vi "Main.vi"(11 "Module Admin":refnum<class "Delacor_lib_QMH_Module Admin.lvclass">) -> ()   [LabVIEW 2018, in "Configuration.lvlib"]
doc: "This template is based off of the Queued Message Handler design pattern and the Queued Message Handler project template that ships with LabVIEW.\n\nThe main difference is that the queue is private to this module and communication between modules is performed via Broadcast and Request events.\n\nRequest events are wrapped in public API methods and are handled in the Event Handling Loop (EHL) of this VI. Any module can register for Broadcast events sent by this module. The EHL generates messages based on user interface actions.\n\nThe Message Handling Loop (MHL) processes messages generated by the EHL, or by other messages. The messages are string values, so new messages can be added easily to the Message Cases case structure in the MHL. Each message cluster can also provide an optional value for Message Data, which is a variant that can be converted to whatever message-specific data is required.\n_____\nBased on DQMH Project Template 6.0.0.91."
uses:
  Configuration.lvlib
  <vilib>/Delacor/Delacor QMH/Libraries/Module Admin_class/Delacor_lib_QMH_Module Admin.lvclass
  Module Data--cluster.ctl
  <vilib>/Delacor/Delacor QMH/Libraries/Message Queue_class/Delacor_lib_QMH_Message Queue.lvclass/Delacor_lib_QMH_Message Queue.ctl
  Stop Argument--cluster.ctl
  <vilib>/Delacor/Delacor QMH/Libraries/Module Admin_class/Delacor_lib_QMH_Module Admin.lvclass/Delacor_lib_QMH_Module Admin.ctl
  <vilib>/Utility/miscctls.llb/LVPointTypeDef.ctl
  <vilib>/Delacor/Delacor QMH/Libraries/Message Queue_class/Delacor_lib_QMH_Enqueue Message (Single).vi
  <vilib>/Delacor/Delacor QMH/Libraries/Module Admin_class/Delacor_lib_QMH_Get External Launch.vi
  <vilib>/Utility/error.llb/Error Cluster From Error Code.vi
  <vilib>/ErrorRing/Error Ring.xnode
  <vilib>/Delacor/Delacor QMH/Libraries/Message Queue_class/Delacor_lib_QMH_Message Queue.lvclass
panel:
  in  "OK":bool
  in  "Cancel":bool
  in  "# DUTs":string
  in  "ma SAP":string
  in  "Password":string
  in  "User":string
  out "error out":errorcluster
  out "Status":string
  in  "Simulate MHL Error":bool
  in  "Simulate EHL Error":bool
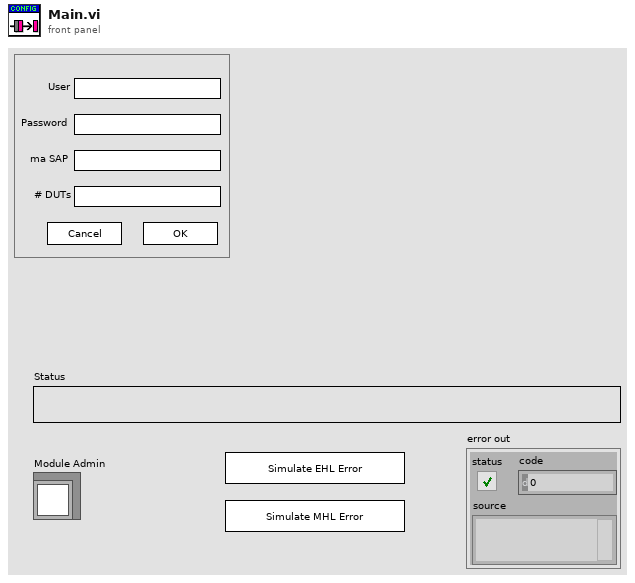
[diagram p1: front panel]
types:
  T1 = enum8{"Enabled", "Disabled", "Disabled and Grayed Out"}
  T2 = typedef "Configuration.lvlib/Request Events--cluster.ctl" = cluster{"Stop Module":refnum<user-event>, "Show Panel":refnum<user-event>, "Hide Panel":refnum<user-event>, "Get Module Execution Status":refnum<user-event>, "Show Diagram":refnum<user-event>}
  T3 = typedef "Configuration.lvlib/Module Data--cluster.ctl" = cluster{"Status":string}
  T4 = enum32{"invalid lock state", "Not Locked", "Locked (No Password)", "Password-protected"}
  T5 = typedef "Configuration.lvlib/Stop Argument--cluster.ctl" = cluster{"Origin":string, "Exit via Stop Module Req?":bool, "Wait for Module to stop?":bool}
  T6 = typedef "LVPointTypeDef.ctl" = cluster{"Horizontal":i16, "Vertical":i16}
  T7 = enum32{"Invalid", "Standard", "Closed", "Hidden", "Minimized", "Maximized"}
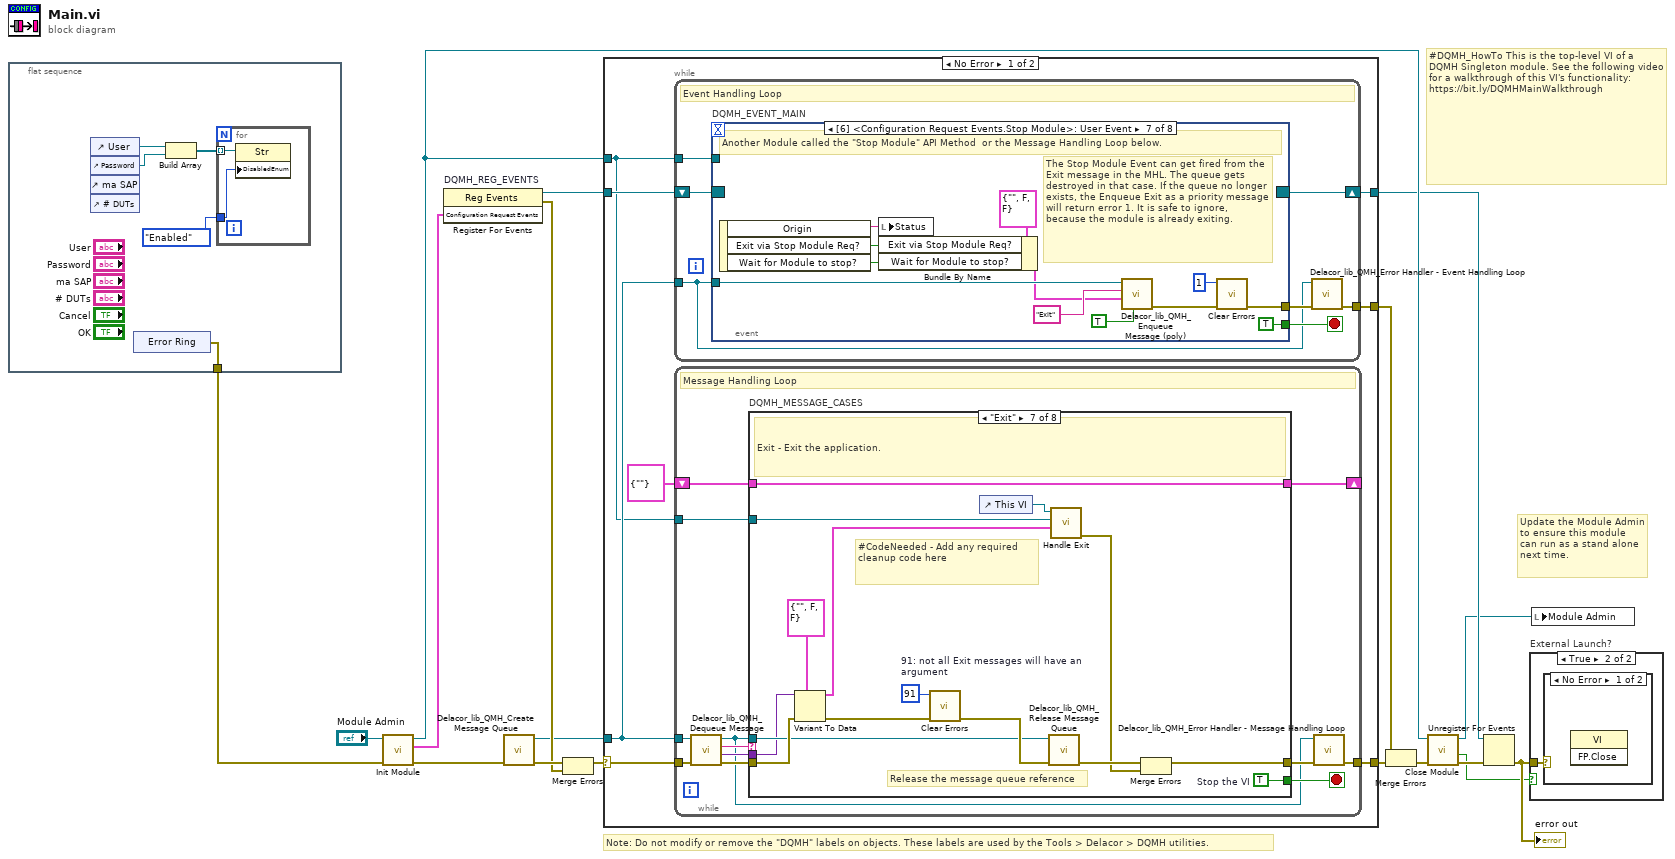
[diagram p0: block diagram]
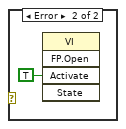
[diagram p3: hidden frame]
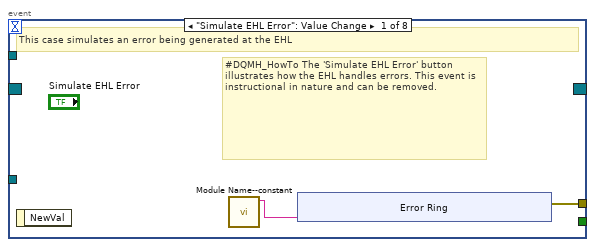
[diagram p4: hidden frame]
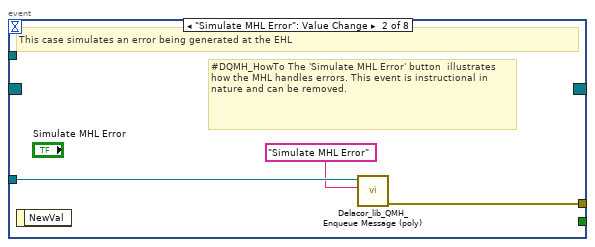
[diagram p5: hidden frame]
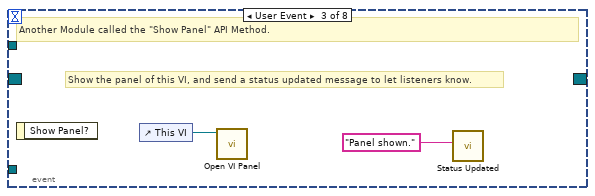
[diagram p6: hidden frame]
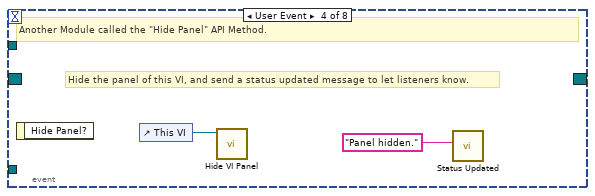
[diagram p7: hidden frame]
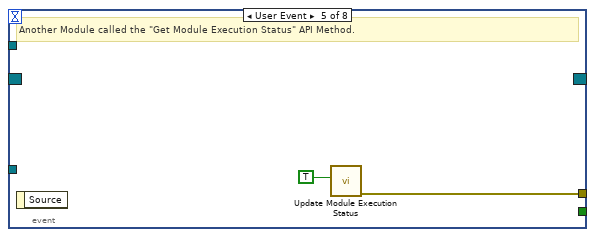
[diagram p8: hidden frame]
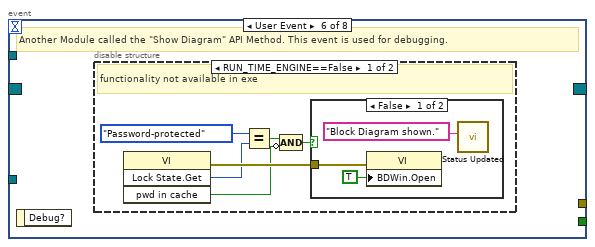
[diagram p9: hidden frame]
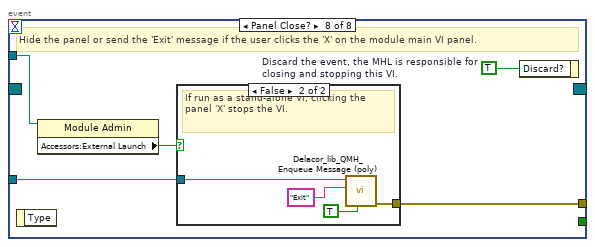
[diagram p12: hidden frame]
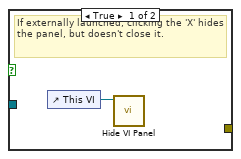
[diagram p13: hidden frame]
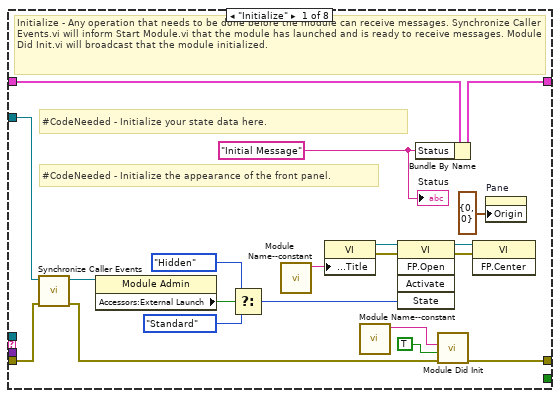
[diagram p14: hidden frame]
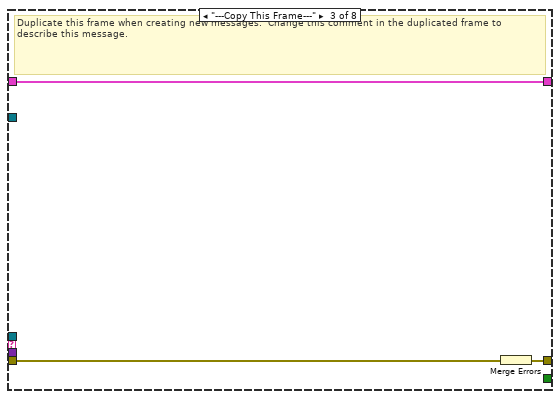
[diagram p16: hidden frame]
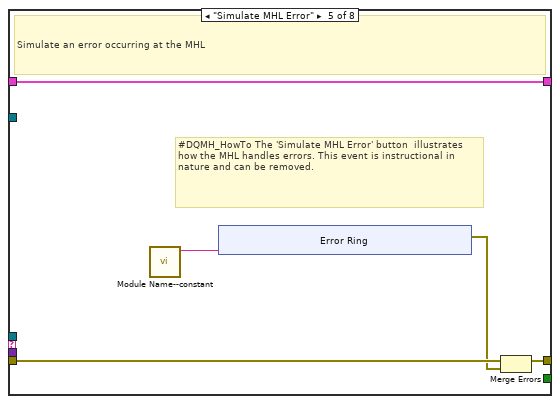
[diagram p18: hidden frame]
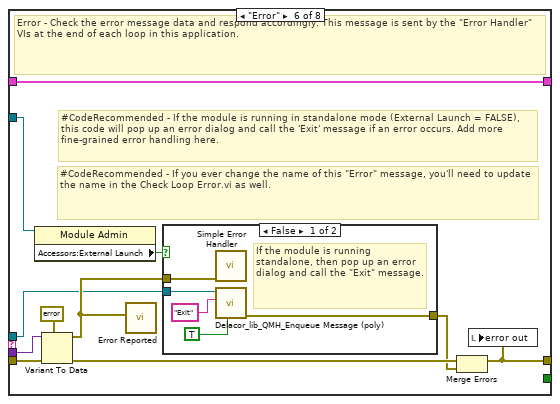
[diagram p19: hidden frame]
diagram:
  # "#DQMH_HowTo This is the top-level VI of a DQMH Singleton module. See the following video for a walkthrough of this VI's functionality: https://bit.ly/DQMHMainWalkthrough"
  # "Note: Do not modify or remove the \"DQMH\" labels on objects. These labels are used by the Tools > Delacor > DQMH utilities."
  # "Update the Module Admin to ensure this module can run as a stand alone next time."
  n1 = flat-sequence {
    tunnel: [w19] -> w1
    frame #0 {
      n2 = control-ref of="User"() -> (w22:refnum<vi>)
      n3 = control-ref of="Password"() -> (w21:refnum<vi>)
      n4 = control-ref of="ma SAP"() -> ()  [unwired: 1 out]
      n5 = control-ref of="# DUTs"() -> ()  [unwired: 1 out]
      n6 = xnode "Error Ring"() -> ("error out"=w19:errorcluster)
      n7 = Build Array(w22, w21) -> (w20:refnum<vi>[])
      n8 = for {
        tunnel: w20 -> [w26] mode=indexing
        tunnel: T1."Enabled" ("Disabled") -> [w25]
        n9 = property class="Str"(reference=w26, "DisabledEnum"=w25) -> ()  [unwired: 1 in, 2 out]
      }
    }
  }
  n10 = call "Init Module.vi"("error in (no error)"=w1, "Singleton Module Admin in"="Module Admin") -> ("error out"=w17:errorcluster, "Configuration Request Events"=w6:T2, "Singleton Module Admin out"=w9:refnum<class "Delacor_lib_QMH_Module Admin.lvclass">)  [unwired: 7 in]
  n11 = register-events "DQMH_REG_EVENTS"(w6) -> (reference out=w7:refnum<event-registration>, error out=w10:errorcluster)  [unwired: 2 in]
  n12 = call <vilib>:"Delacor_lib_QMH_Create Message Queue.vi"("error in"=w17) -> ("error out"=w12:errorcluster, "Message Queue"=w5:refnum<class "Delacor_lib_QMH_Message Queue.lvclass">)  [unwired: 9 in]
  n13 = Merge Errors(w12, w10) -> (w11:errorcluster)
  n14 = case shown="No Error" w11 {
    selector: w11 -> [w32 w189]
    tunnel: [w34 w188] -> w18
    tunnel: [w31 w194] -> w8
    tunnel: w7 -> [w29 w194]
    tunnel: w5 -> [w28 w187]
    tunnel: [w33 _] -> w15
    tunnel: w9 -> [w27 w190]
    frame No Error {
      n15 = while {
        tunnel: w28 -> [w35]
        shift-right: [w38] -> w31
        shift-left: w29 -> [w39]
        tunnel: [w40] -> w33
        tunnel: w27 -> [w36]
        stop <- w37 stop-if-true
        # "Event Handling Loop"
        n16 = event "DQMH_EVENT_MAIN" shown="[6] <Configuration Request Events.Stop Module>: User Event" {
          selector: w39 -> [_ _ _ _ _ _ _ _]
          dyn-events: [_ _ _ _ _ _ _ _] -> w38
          timeout: _ -> [_ _ _ _ _ _ _ _]
          tunnel: [_ _ _ _ _ _ TRUE ("Discard?") _] -> w37
          tunnel: w35 -> [_ w52 _ _ _ _ w76 w83]
          tunnel: [w43 w53 _ _ w59 _ w79 w85] -> w41
          tunnel: w36 -> [_ _ _ _ _ _ _ w82]
          event "Simulate EHL Error": Value Change {
            # "#DQMH_HowTo The 'Simulate EHL Error' button  illustrates how the EHL handles errors. This event is instructional in nature and can be removed."
            # "This case simulates an error being generated at the EHL"
            n17 = event-data() -> ()  [unwired: 1 in, 1 out]
            n18 = call "Module Name--constant.vi"() -> ("Module Name"=w42:string)  [unwired: 11 in]
            n19 = xnode "Error Ring"("parameter 0"=w42) -> ("error out"=w43:errorcluster)
          }
          event "Simulate MHL Error": Value Change {
            # "#DQMH_HowTo The 'Simulate MHL Error' button  illustrates how the MHL handles errors. This event is instructional in nature and can be removed."
            # "This case simulates an error being generated at the EHL"
            n20 = event-data() -> ()  [unwired: 1 in, 1 out]
            n21 = call-poly <vilib>:"Delacor_lib_QMH_Enqueue Message (poly).vi"("Message"="Simulate MHL Error", "Message Queue in"=w52) -> ("error out"=w53:errorcluster)  [unwired: 8 in, 1 out]
          }
          event User Event {
            # "Show the panel of this VI, and send a status updated message to let listeners know."
            # "Another Module called the \"Show Panel\" API Method."
            n22 = event-data() -> ()  [unwired: 1 in, 1 out]
            n23 = control-ref of="This VI"() -> (w55:refnum<vi>)
            n24 = call "Open VI Panel.vi"("VI"=w55) -> ()  [unwired: 10 in, 1 out]
            n25 = call "Status Updated.vi"("Status"="Panel shown." ("format string")) -> ()  [unwired: 10 in, 1 out]
          }
          event User Event {
            # "Hide the panel of this VI, and send a status updated message to let listeners know."
            # "Another Module called the \"Hide Panel\" API Method."
            n26 = event-data() -> ()  [unwired: 1 in, 1 out]
            n27 = control-ref of="This VI"() -> (w57:refnum<vi>)
            n28 = call "Hide VI Panel.vi"("VI"=w57) -> ()  [unwired: 10 in, 1 out]
            n29 = call "Status Updated.vi"("Status"="Panel hidden." ("format string")) -> ()  [unwired: 10 in, 1 out]
          }
          event User Event {
            # "Another Module called the \"Get Module Execution Status\" API Method."
            n30 = event-data() -> ()  [unwired: 1 in, 1 out]
            n31 = call "Update Module Execution Status.vi"("Running?"=TRUE) -> ("error out"=w59:errorcluster)  [unwired: 10 in]
          }
          event User Event {
            # "Another Module called the \"Show Diagram\" API Method. This event is used for debugging."
            n32 = event-data() -> ()  [unwired: 1 in, 1 out]
            n33 = disable-structure shown="RUN_TIME_ENGINE==False" {
              frame condition #0 (active) {
                # "functionality not available in exe"
                n34 = invoke class="VI" method="Lock State.Get"() -> (error out=w65:errorcluster, "Get Lock State"=w64:T4, "pwd in cache"=w61:bool)  [unwired: 4 in, 1 out]
                n35 = Equal?(x=T4."Password-protected", y=w64) -> (x = y?=w62:bool)
                n36 = Compound Arithmetic op=AND(w62, invert w61) -> (w60:bool)
                n37 = case shown="False" w60 {
                  tunnel: w65 -> [w68 _]
                  frame False {
                    n38 = property class="VI"(error in=w68, "BDWin.Open"=TRUE ("Block Diagram Window:Open")) -> ()  [unwired: 1 in, 2 out]
                    n39 = call "Status Updated.vi"("Status"="Block Diagram shown." ("format string")) -> ()  [unwired: 10 in, 1 out]
                  }
                  frame True {
                    # "Password-protected VI, and the password is not in the cache. Do not show the diagram."
                  }
                }
              }
              frame condition #1 {
              }
            }
          }
          event User Event {
            # "The Stop Module Event can get fired from the Exit message in the MHL. The queue gets destroyed in that case. If the queue no longer exists, the Enqueue Exit as a priority message will return error 1. It is safe to ignore, because the module is already exiting."
            # "Another Module called the \"Stop Module\" API Method  or the Message Handling Loop below."
            n40 = event-data() -> ("Origin"=w75:string, "Exit via Stop Module Req?"=w71:bool, "Wait for Module to stop?"=w70:bool)  [unwired: 1 in]
            n41 = local write "Status"(w75) -> ()
            n42 = Bundle By Name(cluster=T5 {"Origin"="", "Exit via Stop Module Req?"=FALSE, "Wait for Module to stop?"=FALSE} ("Stop Argument"), "Exit via Stop Module Req?"=w71, "Wait for Module to stop?"=w70) -> (w69:T5)
            n43 = call-poly <vilib>:"Delacor_lib_QMH_Enqueue Message (poly).vi"("Priority Message? (F)"=TRUE, "Message Data"=w69, "Message"="Exit", "Message Queue in"=w76) -> ("error out"=w80:errorcluster)  [unwired: 6 in, 1 out]
            n44 = call <vilib>:"Clear Errors.vi"("error in (no error)"=w80, "specific error code to clear (0: all)"=1) -> ("error out"=w79:errorcluster)  [unwired: 4 in, 1 out]
          }
          event Panel Close? {
            w84 = TRUE  # Discard the event, the MHL is responsible for closing and stopping this VI.
            # "Hide the panel or send the 'Exit' message if the user clicks the 'X' on the module main VI panel."
            n45 = event-data() -> ()  [unwired: 1 in, 1 out]
            n46 = property class="Module Admin"(reference=w82) -> ("Accessors:External Launch"=w81:bool)  [unwired: 1 in, 2 out]
            n47 = case shown="False" w81 {
              tunnel: w83 -> [_ w89]
              tunnel: [_ w90] -> w85
              frame True {
                # "If externally launched, clicking the 'X' hides the panel, but doesn't close it."
                n48 = control-ref of="This VI"() -> (w86:refnum<vi>)
                n49 = call "Hide VI Panel.vi"("VI"=w86) -> ()  [unwired: 10 in, 1 out]
              }
              frame False {
                # "If run as a stand-alone VI, clicking the panel 'X' stops the VI."
                n50 = call-poly <vilib>:"Delacor_lib_QMH_Enqueue Message (poly).vi"("Priority Message? (F)"=TRUE, "Message"="Exit", "Message Queue in"=w89) -> ("error out"=w90:errorcluster)  [unwired: 7 in, 1 out]
              }
            }
            n51 = event-data("Discard?"=w84) -> ()  [unwired: 1 in, 1 out]
          }
        }
        n52 = call-dynamic "Delacor_lib_QMH_Error Handler - Event Handling Loop.vi"("error in"=w41, "Message Queue in"=w35) -> ("dup error in"=w40:errorcluster)  [unwired: 8 in, 1 out]
      }
      n53 = while {
        tunnel: w28 -> [w93]
        shift-right: [w97] -> _
        shift-left: T3 {"Status"=""} ("Data Cluster") -> [w98]
        tunnel: w32 -> [w101]
        tunnel: [w99] -> w34
        tunnel: w27 -> [w91]
        stop <- w96 stop-if-true
        # "Message Handling Loop"
        n54 = call-dynamic "Delacor_lib_QMH_Dequeue Message.vi"("error in"=w101, "Message Queue in"=w93) -> ("error out"=w100:errorcluster, "Message Data"=w94:variant, "Message"=w95:string, "Message Queue out"=w92:refnum<class "Delacor_lib_QMH_Message Queue.lvclass">)  [unwired: 6 in]
        n55 = case "DQMH_MESSAGE_CASES" shown="\"Exit\"" w95 {
          selector: w95 -> [_ _ _ _ _ _ _ w174]
          tunnel: w92 -> [_ _ _ _ _ w144 w166 _]
          tunnel: w100 -> [w120 w124 w127 w129 w134 w151 w172 w176]
          tunnel: [w118 w124 w126 w129 w133 w147 w169 w177] -> w102
          tunnel: w98 -> [w109 w123 w125 w128 w131 w146 w165 w175]
          tunnel: [w108 w123 w125 w128 w131 w146 w165 w175] -> w97
          tunnel: [_ _ _ _ _ _ w164 _] -> w96
          tunnel: w94 -> [_ _ _ _ _ w145 w163 _]
          tunnel: w91 -> [w110 _ _ _ _ w143 w158 _]
          frame "Initialize" {
            w104 = "Initial Message" ("Initial Message")
            # "#CodeNeeded - Initialize the appearance of the front panel."
            # "#CodeNeeded - Initialize your state data here."
            # "Initialize - Any operation that needs to be done before the module can receive messages. Synchronize Caller Events.vi will inform Start Module.vi that the module has launched and is ready to receive messages. Module Did Init.vi will broadcast that the module initialized."
            n56 = call "Synchronize Caller Events.vi"("error in (no error)"=w120, "Singleton Module Admin in"=w110) -> ("error out"=w119:errorcluster, "Singleton Module Admin out"=w105:refnum<class "Delacor_lib_QMH_Module Admin.lvclass">)  [unwired: 8 in]
            n57 = property class="Module Admin"(reference=w105) -> ("Accessors:External Launch"=w114:bool)  [unwired: 1 in, 2 out]
            n58 = Select(t=T7."Hidden" ("State"), s=w114, f=T7."Standard" ("State")) -> (s? t:f=w111:T7)
            n59 = call "Module Name--constant.vi"() -> ("Module Name"=w117:string)  [unwired: 11 in]
            n60 = property class="VI"("Front Panel.Title"=w117) -> (reference out=w116:refnum<vi>, error out=w122:errorcluster)  [unwired: 2 in]
            n61 = call "Module Name--constant.vi"() -> ("Module Name"=w106:string)  [unwired: 11 in]
            n62 = invoke class="VI" method="FP.Open"(reference=w116, error in=w122, "State"=w111) -> (reference out=w115:refnum<vi>, error out=w121:errorcluster)  [unwired: 2 in, 3 out]
            n63 = Bundle By Name(cluster=w109, "Status"=w104) -> (w108:T3)
            n64 = call "Module Did Init.vi"("error in (no error)"=w119, "Initialized?"=TRUE, "Origin"=w106) -> ("error out"=w118:errorcluster)  [unwired: 8 in]
            n65 = invoke class="VI" method="FP.Center"(reference=w115, error in=w121) -> ()  [unwired: 1 in, 3 out]
            n66 = property on="Pane" class="Pane"("Origin"=T6 {"Horizontal"=0, "Vertical"=0}) -> ()  [unwired: 2 in, 2 out]
            "Status" <- w104
          }
          frame "---Module Specific---" {
            # "Separator -- The following cases handle messages specific to this Module."
          }
          frame "---Copy This Frame---" {
            # "Duplicate this frame when creating new messages.  Change this comment in the duplicated frame to describe this message."
            n67 = Merge Errors(w127) -> (w126:errorcluster)
          }
          frame "---Exit and Error Handling---" {
            # "Separator - The following cases handle errors and exit messages."
          }
          frame "Simulate MHL Error" {
            # "#DQMH_HowTo The 'Simulate MHL Error' button  illustrates how the MHL handles errors. This event is instructional in nature and can be removed."
            # "Simulate an error occurring at the MHL"
            n68 = call "Module Name--constant.vi"() -> ("Module Name"=w130:string)  [unwired: 11 in]
            n69 = xnode "Error Ring"("parameter 0"=w130) -> ("error out"=w132:errorcluster)
            n70 = Merge Errors(w134, w132) -> (w133:errorcluster)
          }
          frame "Error" {
            # "#CodeRecommended - If you ever change the name of this \"Error\" message, you'll need to update the name in the Check Loop Error.vi as well."
            # "#CodeRecommended - If the module is running in standalone mode (External Launch = FALSE), this code will pop up an error dialog and call the 'Exit' message if an error occurs. Add more fine-grained error handling here."
            # "Error - Check the error message data and respond accordingly. This message is sent by the \"Error Handler\" VIs at the end of each loop in this application."
            n71 = property class="Module Admin"(reference=w143) -> ("Accessors:External Launch"=w142:bool)  [unwired: 1 in, 2 out]
            n72 = Variant To Data(error in=w151, type=errorcluster {"status"=FALSE, "code"=0, "source"=""} ("error constant"), Variant=w145) -> (data=w152:errorcluster, error out=w149:errorcluster)
            n73 = call "Error Reported.vi"("Error"=w152) -> ()  [unwired: 10 in, 1 out]
            n74 = case shown="False" w142 {
              tunnel: [w157 _] -> w148
              tunnel: w144 -> [w155 _]
              tunnel: w152 -> [w156 _]
              frame False {
                # "If the module is running standalone, then pop up an error dialog and call the \"Exit\" message."
                n75 = call <vilib>:"Simple Error Handler.vi"("error in (no error)"=w156) -> ()  [unwired: 4 in, 5 out]
                n76 = call-poly <vilib>:"Delacor_lib_QMH_Enqueue Message (poly).vi"("Priority Message? (F)"=TRUE, "Message"="Exit", "Message Queue in"=w155) -> ("error out"=w157:errorcluster)  [unwired: 7 in, 1 out]
              }
              frame True {
                # "If the module was launched externally, calling the Error Reported broadcast VI is the only action performed by the \"Error\" message. The module's caller can then process the error appropriately."
              }
            }
            n77 = Merge Errors(w149, w148) -> (w147:errorcluster)
            n78 = local write "error out"(w147) -> ()
          }
          frame "Exit" {
            w162 = 91  # 91: not all Exit messages will have an argument
            w164 = TRUE  # Stop the VI
            # "Release the message queue reference"
            # "#CodeNeeded - Add any required cleanup code here"
            # "Exit - Exit the application."
            n79 = Variant To Data(error in=w172, type=T5 {"Origin"="", "Exit via Stop Module Req?"=FALSE, "Wait for Module to stop?"=FALSE} ("Stop Argument"), Variant=w163) -> (data=w160:T5, error out=w168:errorcluster)
            n80 = call <vilib>:"Clear Errors.vi"("error in (no error)"=w168, "specific error code to clear (0: all)"=w162) -> ("error out"=w171:errorcluster)  [unwired: 4 in, 1 out]
            n81 = control-ref of="This VI"() -> (w159:refnum<vi>)
            n82 = call-dynamic "Delacor_lib_QMH_Release Message Queue.vi"("error in"=w171, "Message Queue"=w166) -> ("error out"=w170:errorcluster)  [unwired: 9 in]
            n83 = call "Handle Exit.vi"("Stop Argument"=w160, "Admin in"=w158, "VI reference"=w159) -> ("error out"=w167:errorcluster)  [unwired: 7 in, 1 out]
            n84 = Merge Errors(w170, w167) -> (w169:errorcluster)
          }
          frame Default {
            # "'Default' case only runs if there is a message that isn't defined in any of the other cases.  Output a programming error."
            n85 = call "Module Name--constant.vi"() -> ("Module Name"=w173:string)  [unwired: 11 in]
            n86 = xnode "Error Ring"("parameter 0"=w174, "parameter 1"=w173) -> ("error out"=w178:errorcluster)
            n87 = Merge Errors(w176, w178) -> (w177:errorcluster)
          }
        }
        n88 = call-dynamic "Delacor_lib_QMH_Error Handler - Message Handling Loop.vi"("error in"=w102, "Message Queue in"=w92) -> ("dup error in"=w99:errorcluster)  [unwired: 8 in, 1 out]
      }
    }
    frame Error {
      # "Synchronize Caller Events.vi will inform Start Module.vi that the module has launched and will let the code calling Start Module.vi register for broadcasts and would permit the caller receive the broadcast that an error occurred at launch time."
      n89 = call-dynamic "Delacor_lib_QMH_Release Message Queue.vi"("error in"=w189, "Message Queue"=w187) -> ("error out"=w188:errorcluster)  [unwired: 9 in]
      n90 = call "Synchronize Caller Events.vi"("Singleton Module Admin in"=w190) -> ("error out"=w195:errorcluster)  [unwired: 9 in, 1 out]
      n91 = call "Module Name--constant.vi"() -> ("Module Name"=w193:string)  [unwired: 11 in]
      n92 = Format Into String(format string="An error occurred during initialization. %s is no longer running.", w193) -> (resulting string=w191:string)  [unwired: 2 in, 1 out]
      n93 = Merge Errors(w188, w195) -> (w196:errorcluster)
      n94 = call "Error Reported.vi"("Additional Information"=w191, "Error"=w196) -> ()  [unwired: 9 in, 1 out]
    }
  }
  n95 = Merge Errors(w15, w18) -> (w14:errorcluster)
  n96 = call "Close Module.vi"("error in (no error)"=w14, "Module Admin in"=w9) -> ("error out"=w16:errorcluster, "External Launch"=w2:bool, "Module Admin out"=w3:refnum<class "Delacor_lib_QMH_Module Admin.lvclass">)  [unwired: 7 in]
  n97 = Unregister For Events(event registration refnum=w8, error in=w16) -> (error out=w13:errorcluster)
  "error out" <- w13
  n98 = case "External Launch?" shown="True" w2 {
    tunnel: w13 -> [_ w197]
    frame False {
    }
    frame True {
      n99 = case shown="No Error" w197 {
        frame No Error {
          n100 = invoke class="VI" method="FP.Close"() -> ()  [unwired: 3 in, 3 out]
        }
        frame Error {
          n101 = invoke class="VI" method="FP.Open"("Activate"=TRUE ("Activate?")) -> ()  [unwired: 4 in, 5 out]
        }
      }
    }
  }
  n102 = local write "Module Admin"(w3) -> ()
